vi "Cal BC (Numeric).vi"(8 "error in (no error)":errorcluster, 10 "BC in":variant, 11 "Domain_Evolut_1D in":refnum<class "NI_Domain_Evolut_1D.lvclass">) -> (0 "error out":errorcluster, 2 "BC out":variant, 3 "Domain_Evolut_1D out":refnum<class "NI_Domain_Evolut_1D.lvclass">)   [LabVIEW 2020, in "NI_PDE.lvlib" / "NI_Domain_Evolut_1D.lvclass"]
uses:
  <vilib>/gmath/pde.llb/DomainClass/Domain_Evolut_1D/NI_Domain_Evolut_1D.lvclass
  <vilib>/gmath/pde.llb/BCClass/BC_Evolut_1D_Numeric/BC Data.ctl
  <vilib>/gmath/pde.llb/Common/PDE_BC Type.ctl
  <vilib>/gmath/pde.llb/Common/PDE_BC Position 1D.ctl
  <vilib>/gmath/NI_PDE.lvlib
  <vilib>/gmath/pde.llb/BCClass/BC_Evolut_1D_Numeric/NI_BC_Evolut_1D_Numeric.lvclass
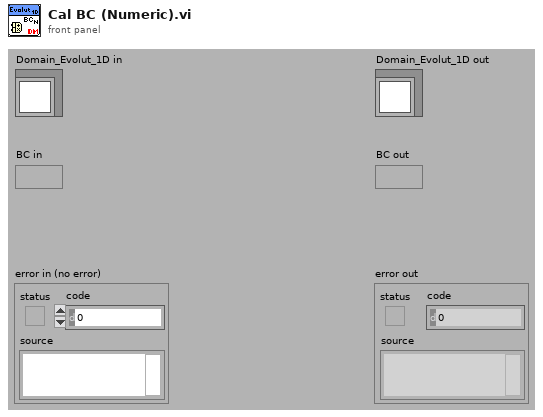
[diagram p1: front panel]
types:
  T1 = typedef "NI_PDE.lvlib/NI_BC_Evolut_1D_Numeric.lvclass/BC Data.ctl" = cluster{"type":T2, "position":T3, "G":dbl[]}
  T2 = typedef "NI_PDE.lvlib/PDE_BC Type.ctl" = i32
  T3 = typedef "NI_PDE.lvlib/PDE_BC Position 1D.ctl" = i32
  T4 = cluster{"initial t":dbl, "final t":dbl, "# of t-points":i32}
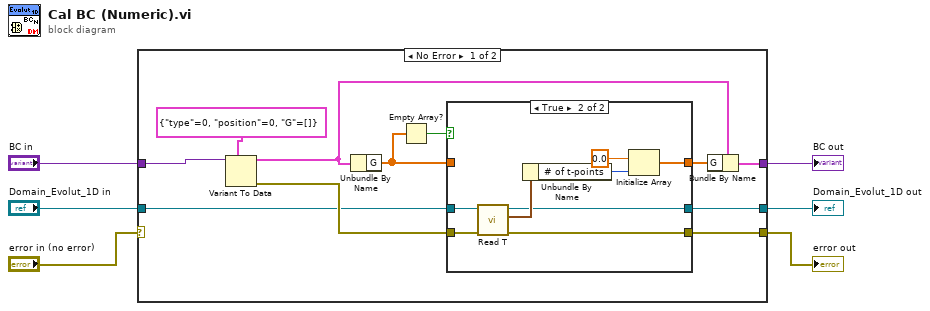
[diagram p0: block diagram]
diagram:
  n1 = case shown="No Error" "error in (no error)" {
    selector: "error in (no error)" -> [_ w31]
    tunnel: "Domain_Evolut_1D in" -> [w13 w30]
    tunnel: [w8 w30] -> w6
    tunnel: [w7 w31] -> w5
    tunnel: [w9 w29] -> w2
    tunnel: "BC in" -> [w16 w29]
    frame No Error {
      n2 = Variant To Data(type=T1 {"type"=0, "position"=0, "G"=[]} ("BC data"), Variant=w16) -> (data=w11:T1, error out=w14:errorcluster)  [unwired: 1 in]
      n3 = Unbundle By Name(w11) -> ("G"=w12:dbl[])
      n4 = Empty Array?(array=w12) -> (empty?=w17:bool)
      n5 = case shown="True" w17 {
        tunnel: w13 -> [w18 w23]
        tunnel: w14 -> [w19 w22]
        tunnel: w12 -> [w20 _]
        tunnel: [w19 w25] -> w7
        tunnel: [w20 w27] -> w10
        tunnel: [w18 w21] -> w8
        frame False {
        }
        frame True {
          n6 = call-dynamic "Read T.vi"("error in (no error)"=w22, "Domain_Evolut.lvclass in"=w23) -> ("error out"=w25:errorcluster, "t"=w28:T4, "Domain_Evolut.lvclass out"=w21:refnum<class "NI_Domain_Evolut_1D.lvclass">)  [unwired: 7 out]
          n7 = Unbundle By Name(w28) -> ("# of t-points"=w24:i32)
          n8 = Initialize Array(0.0 ("element"), w24) -> (w27:dbl[])
        }
      }
      n9 = Bundle By Name(cluster=w11, "G"=w10) -> (w9:T1)
    }
    frame Error {
    }
  }
  "Domain_Evolut_1D out" <- w6
  "error out" <- w5
  "BC out" <- w2
